vi "A_vs_B(SubVI).vi"(11 "Versenyzõk":string[][](array[string])) -> (2 "B csapat versenyzõje":string, 3 "A csapat versenyzõje":string)   [LabVIEW 2013]
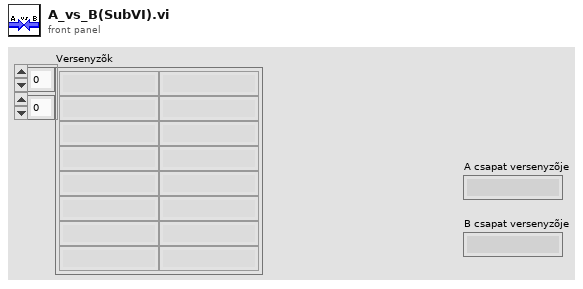
[diagram p1: front panel]
types:
  T1 = cluster{"Versenyzõk[0]":string, "Versenyzõk[1]":string, "Versenyzõk[2]":string, "Versenyzõk[3]":string, "Versenyzõk[4]":string, "Versenyzõk[5]":string, "Versenyzõk[6]":string, "Versenyzõk[7]":string, "Versenyzõk[8]":string}
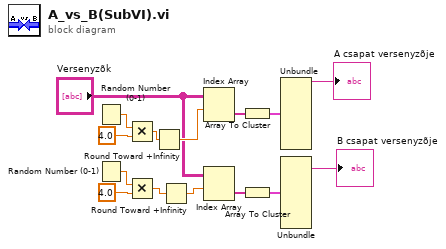
[diagram p0: block diagram]
diagram:
  n1 = Random Number (0-1)() -> (number: 0 to 1=w8:dbl)
  n2 = Random Number (0-1)() -> (number: 0 to 1=w5:dbl)
  n3 = Multiply(x=w8, y=4.0) -> (x*y=w15:dbl)
  n4 = Multiply(x=w5, y=4.0) -> (x*y=w12:dbl)
  n5 = Round Toward +Infinity(x=w15) -> (ceil(x): smallest int >= x=w14:dbl)
  n6 = Round Toward +Infinity(x=w12) -> (ceil(x): smallest int >= x=w13:dbl)
  n7 = Index Array(array="Versenyzõk", index (row)=w14) -> (element=w7:string[])  [unwired: 1 in]
  n8 = Index Array(array="Versenyzõk", index (row)=w13) -> (element=w6:string[])  [unwired: 1 in]
  n9 = Array To Cluster(array=w7) -> (cluster=w10:T1)
  n10 = Array To Cluster(array=w6) -> (cluster=w3:T1)
  n11 = Unbundle(w10) -> ("Versenyzõk[0]"=→"A csapat versenyzõje":string)  [unwired: 8 out]
  n12 = Unbundle(w3) -> ("Versenyzõk[1]"=→"B csapat versenyzõje":string)  [unwired: 8 out]
